vi "Do.vi"(8 "error in (no error)":errorcluster, 10 "Actor in":refnum<class "Actor.lvclass">, 11 "Update Pump State Msg":refnum<class "Update Pump State Msg.lvclass">) -> (0 "error out":errorcluster, 2 "Actor out":refnum<class "Actor.lvclass">)   [LabVIEW 2018, in "Evaporative Cooler Controller.lvlib" / "Update Pump State Msg.lvclass"]
uses:
  Update Pump State Msg.lvclass
  <vilib>/ActorFramework/Actor/Actor.lvclass
  Evaporative Cooler Controller/Evaporative Cooler Controller.lvclass
  C:/Program Files (x86)/National Instruments/LabVIEW 2018/vi.lib/ActorFramework/Actor/Actor.lvclass
  Update Pump State Msg.lvclass/Update Pump State Msg.ctl
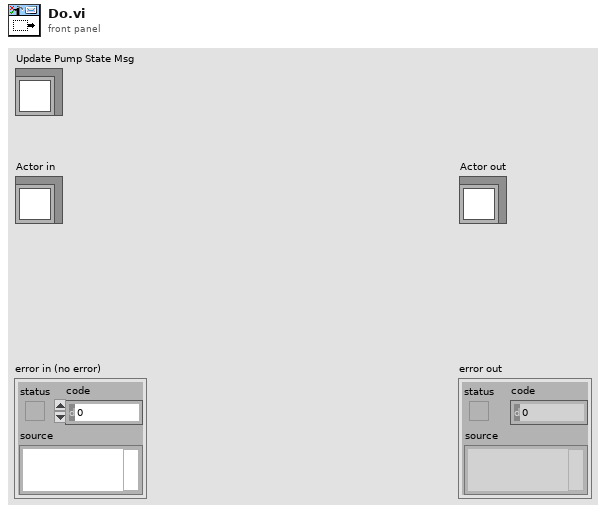
[diagram p1: front panel]
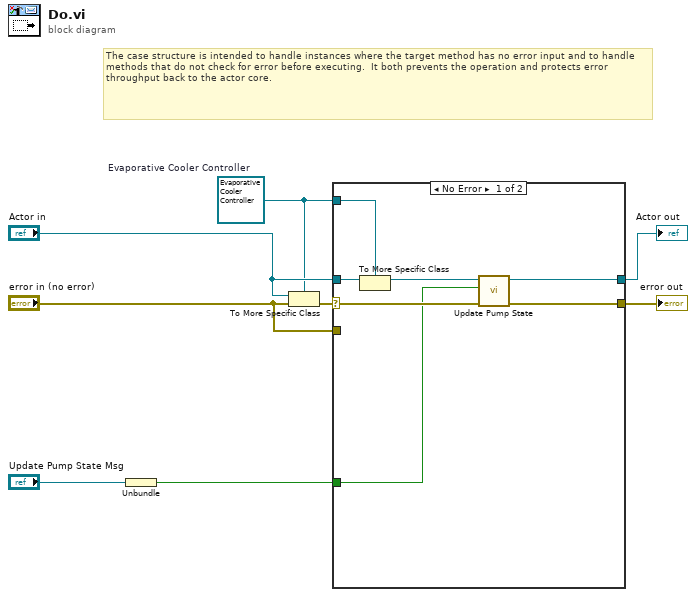
[diagram p0: block diagram]
diagram:
  w3 = refnum<class "Evaporative Cooler Controller.lvclass"> refnum  # Evaporative Cooler Controller
  # "The case structure is intended to handle instances where the target method has no error input and to handle methods that do not check for error before executing.  It both prevents the operation and protects error throughput back to the actor core."
  n1 = Unbundle("Update Pump State Msg") -> (w2:bool)
  n2 = To More Specific Class(target class=w3, reference="Actor in", error in="error in (no error)") -> (error out=w7:errorcluster)  [unwired: 1 out]
  n3 = case shown="No Error" w7 {
    selector: w7 -> [w13 _]
    tunnel: [w15 w16] -> w6
    tunnel: [w14 w17] -> w5
    tunnel: "Actor in" -> [w12 w17]
    tunnel: w3 -> [w11 _]
    tunnel: w2 -> [w9 _]
    tunnel: "error in (no error)" -> [_ w16]
    frame No Error {
      n4 = To More Specific Class(target class=w11, reference=w12) -> (specific class reference=w10:refnum<class "Evaporative Cooler Controller.lvclass">)  [unwired: 1 in, 1 out]
      n5 = call-dynamic "Update Pump State.vi"("error in (no error)"=w13, "Pump on?"=w9, "Evaporative Cooler Controller in"=w10) -> ("error out"=w15:errorcluster, "Evaporative Cooler Controller out"=w14:refnum<class "Evaporative Cooler Controller.lvclass">)  [unwired: 7 in]
    }
    frame Error {
      # "This Do.vi looks somewhat different from the standard. Here, we have decided that if this controller is not of the right type, that's ok. We ignore the error from the To More Specific Class function and just silently drop this message. This allows a plain Cooler Controller to control the Evaporative Cooler, even though a plain Cooler Controller has no idea how to handle all the messages coming out of the Evaporative Cooler. Since these are only status messages, we consider that to be ok."
    }
  }
  "error out" <- w6
  "Actor out" <- w5
